vi "WriteVARIABLE_NAME.vi"(8 "error in (no error)":errorcluster, 10 "VARIABLE_NAME":string, 11 "object in":refnum<class "SetIntermediateValue.lvclass">) -> (0 "error out":errorcluster, 3 "object out":refnum<class "SetIntermediateValue.lvclass">)   [LabVIEW 2017, in "SetIntermediateValue.lvclass"]
uses:
  SetIntermediateValue.lvclass
  SetIntermediateValue.lvclass/SetIntermediateValue.ctl
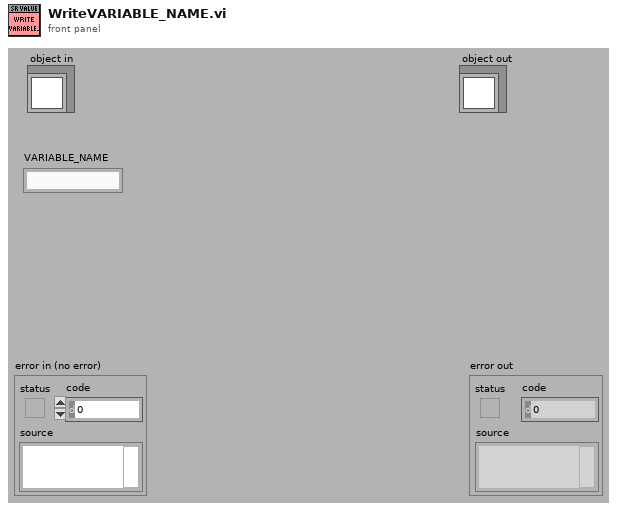
[diagram p1: front panel]
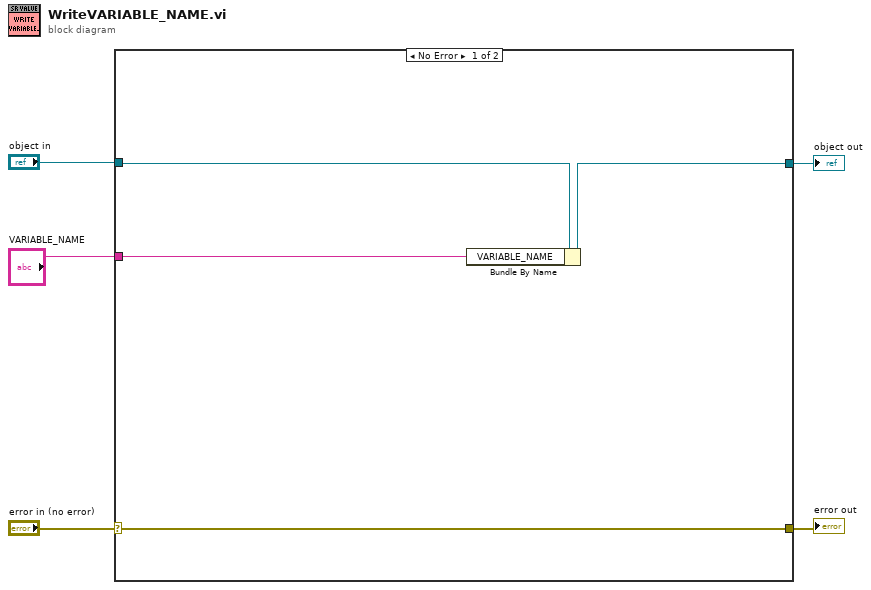
[diagram p0: block diagram]
diagram:
  n1 = case shown="No Error" "error in (no error)" {
    selector: "error in (no error)" -> [w8 w11]
    tunnel: [w8 w11] -> w4
    tunnel: [w6 w10] -> w2
    tunnel: "object in" -> [w7 w10]
    tunnel: "VARIABLE_NAME" -> [w9 _]
    frame No Error {
      n2 = Bundle By Name(cluster=w7, "VARIABLE_NAME"=w9) -> (w6:refnum<class "SetIntermediateValue.lvclass">)
    }
    frame Error {
    }
  }
  "error out" <- w4
  "object out" <- w2
